vi "GET_SD_CARD_INFO.vi"(8 "error in (no error)":errorcluster) -> (0 "error out":errorcluster)   [LabVIEW 2019]
uses:
  Typedefs/Message.ctl
  Typedefs/Sensor Types.ctl
  Typedefs/Message Types.ctl
  Message Globals.vi
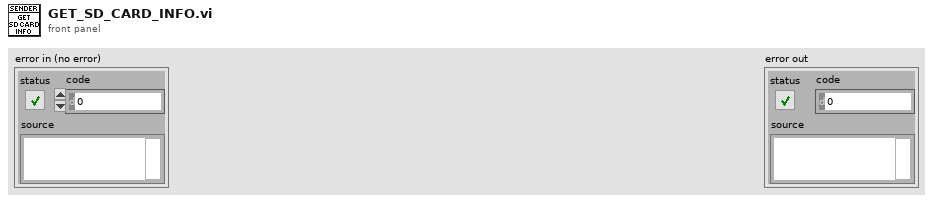
[diagram p1: front panel]
types:
  T1 = typedef "Message Types.ctl" = enum16{"HEART_BEAT", "CONNECT", "GET_CURRENT_MEASUREMENTS", "GET_LOG_FILE", "SEND_LOG_FILE_SIZE", "SEND_LOG_FILE_CHUNK", "GET_LOGGING_PERIOD", "SET_LOGGING_PERIOD", "SEND_SD_CARD_INFO", "GET_LOGS_LIST", "SEND_LOG_FILE_NAME", "SEND_LOGGING_PERIOD", "GET_RTC_TIME", "SET_RTC_TIME", "SEND_RTC_TIME", "SEND_CURRENT_MEASUREMENTS", "DELETE_LOG_FILE", "GET_SD_CARD_INFO", "GET_BATTERY_INFO", "SEND_BATTERY_INFO", "GET_LOG_FILE_SIZE", "ERROR_MSG"}
  T2 = typedef "Message.ctl" = cluster{"Payload Size":u8, "Sequence Number":u8, "Sensor Type":T3, "Message Types":T1, "Data":u8[]}
  T3 = typedef "Sensor Types.ctl" = enum16{"APP", "TURBIDITY", "PH"}
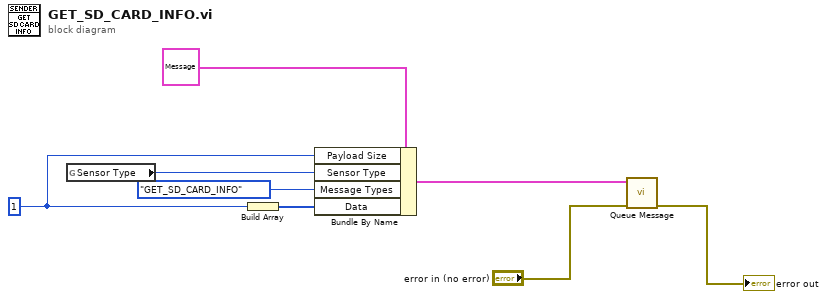
[diagram p0: block diagram]
diagram:
  w1 = u8 1 ("element")
  n1 = global read "Message Globals.vi" "Sensor Type"() -> (w6:T3)
  n2 = Build Array(w1) -> (w2:u8[])
  n3 = Bundle By Name(cluster=T2 {"Payload Size"=0, "Sequence Number"=0, "Sensor Type"=enum."APP", "Message Types"=enum."HEART_BEAT", "Data"=[]} ("Message"), "Payload Size"=w1, "Sensor Type"=w6, "Message Types"=Message_Types."GET_SD_CARD_INFO", "Data"=w2) -> (w5:T2)
  n4 = call "Queue Message.vi"("error in (no error)"="error in (no error)", "Message"=w5) -> ("error out"=→"error out":errorcluster)  [unwired: 9 in]
